vi "trabajo de clase 2.vi"() -> ()   [LabVIEW 2013]
uses:
  <vilib>/express/express arith-compare/Formula/XNode/ExpressFormulaBlockNode.xnode
panel:
  out "abs":string
  in  "Finalizar":bool
  in  "Generar impar":bool
  in  "Generar par":bool
  out "Numero impar":dbl
  out "Numero par":dbl
  # "Usando eventos generar un numero par al presionar un Generar Par\ny generar in numero impar al presionar Generar Impar."
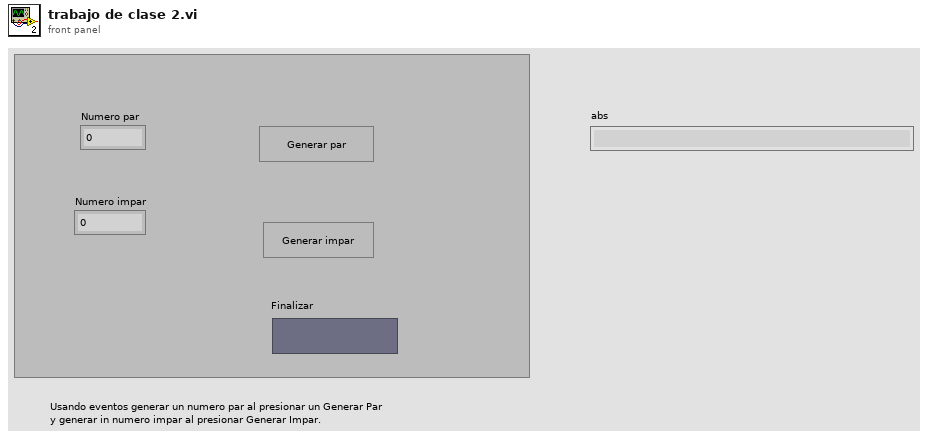
[diagram p1: front panel]
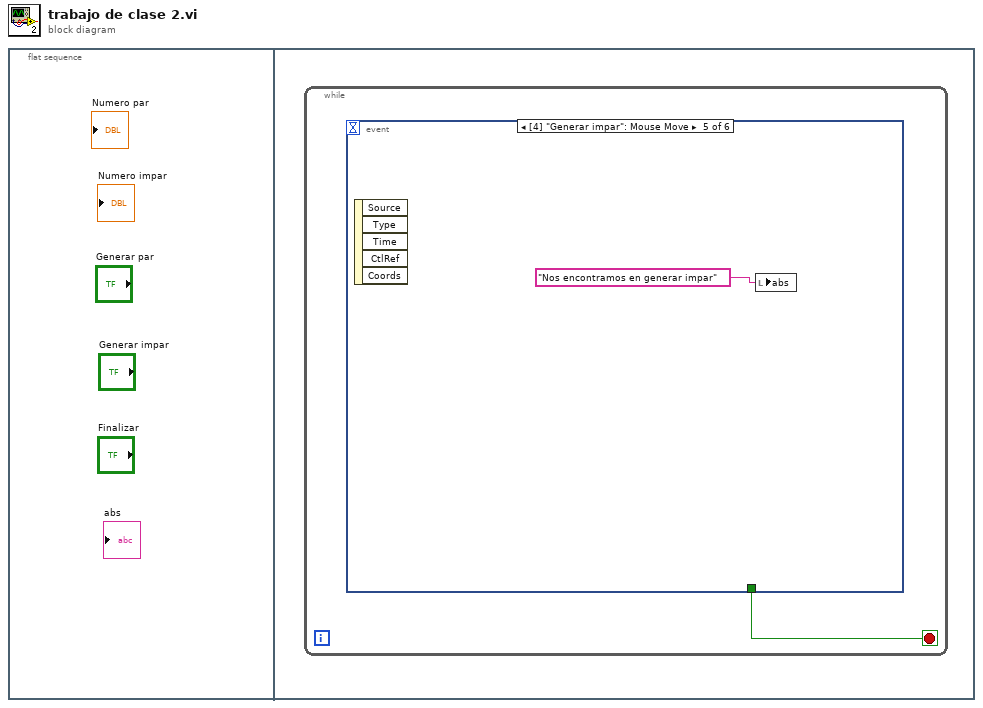
[diagram p0: block diagram]
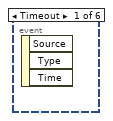
[diagram p2: hidden frame]
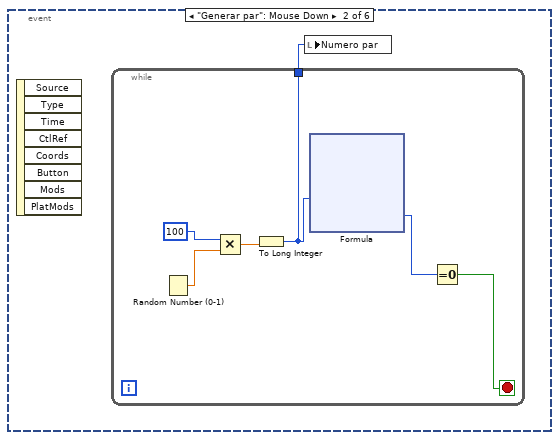
[diagram p3: hidden frame]
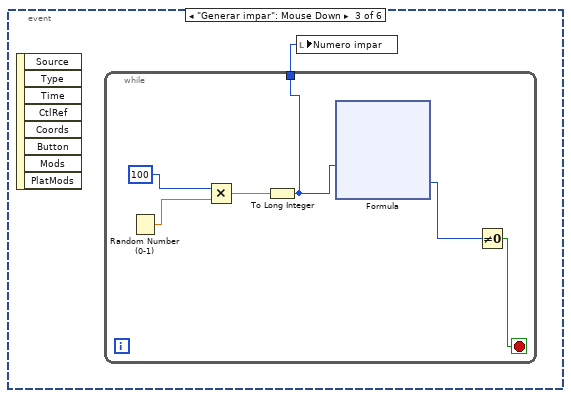
[diagram p4: hidden frame]
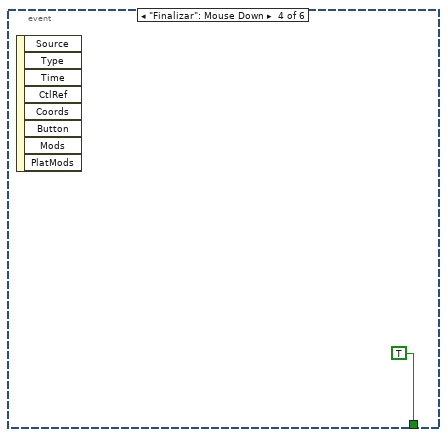
[diagram p5: hidden frame]
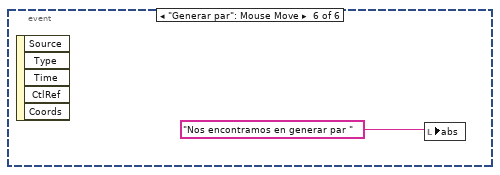
[diagram p6: hidden frame]
diagram:
  n1 = flat-sequence {
    frame #0 {
    }
    frame #1 {
      n2 = while {
        stop <- w1 stop-if-true
        n3 = event shown="[4] \"Generar impar\": Mouse Move" {
          selector: _ -> [_ _ _ _ _ _]
          dyn-events: _ -> [_ _ _ _ _ _]
          timeout: _ -> [_ _ _ _ _ _]
          tunnel: [_ _ _ TRUE _ _] -> w1
          event Timeout {
            n4 = event-data() -> ()  [unwired: 1 in, 3 out]
          }
          event "Generar par": Mouse Down {
            n5 = event-data() -> ()  [unwired: 1 in, 8 out]
            n6 = while {
              tunnel: [w3] -> w2
              stop <- w4 stop-if-true
              n7 = Random Number (0-1)() -> (number: 0 to 1=w6:dbl)
              n8 = Multiply(x=100, y=w6) -> (x*y=w8:dbl)
              n9 = To Long Integer(number=w8) -> (32bit integer=w3:i32)
              n10 = xnode "Formula"("X1"=w3) -> ("Result"=w5:i32)  [unwired: 1 in, 1 out]
              n11 = Equal To 0?(x=w5) -> (x = 0?=w4:bool)
            }
            n12 = local write "Numero par"(w2) -> ()
          }
          event "Generar impar": Mouse Down {
            n13 = event-data() -> ()  [unwired: 1 in, 8 out]
            n14 = while {
              tunnel: [w19] -> w17
              stop <- w18 stop-if-true
              n15 = Random Number (0-1)() -> (number: 0 to 1=w22:dbl)
              n16 = Multiply(x=100, y=w22) -> (x*y=w21:dbl)
              n17 = To Long Integer(number=w21) -> (32bit integer=w19:i32)
              n18 = xnode "Formula"("X1"=w19) -> ("Result"=w20:i32)  [unwired: 1 in, 1 out]
              n19 = Not Equal To 0?(x=w20) -> (x != 0?=w18:bool)
            }
            n20 = local write "Numero impar"(w17) -> ()
          }
          event "Finalizar": Mouse Down {
            n21 = event-data() -> ()  [unwired: 1 in, 8 out]
          }
          event "Generar impar": Mouse Move {
            n22 = event-data() -> ()  [unwired: 1 in, 5 out]
            n23 = local write "abs"("Nos encontramos en generar impar") -> ()
          }
          event "Generar par": Mouse Move {
            n24 = event-data() -> ()  [unwired: 1 in, 5 out]
            n25 = local write "abs"("Nos encontramos en generar par ") -> ()
          }
        }
      }
    }
  }
